vi "Test Default String Output.vi"(8 "error in (no error)":errorcluster) -> (0 "error out":errorcluster)   [LabVIEW 2016, in "UT_Formatter.lvlib"]
doc: "Template for an unit test with caraya in the \"Given, When, Then\" structure from James."
uses:
  UT_Formatter.lvlib
  Source/HSE-Logger/LogLevel.ctl
  Source/HSE-Logger/LogRecord/LogRecord.lvclass/LogRecord.ctl
  <vilib>/addons/_JKI Toolkits/Caraya/classes/Assert/Assert Equal Value_Variant.vi
  Source/HSE-Logger/Formatter/Formatter.lvclass
  <vilib>/addons/_JKI Toolkits/Caraya/classes/Test/Test.lvclass
  <vilib>/addons/_JKI Toolkits/Caraya/classes/Assert/Assert.lvclass
  Source/HSE-Logger/LogRecord/LogRecord.lvclass
  Source/HSE-Logger/hse-logger.lvlib
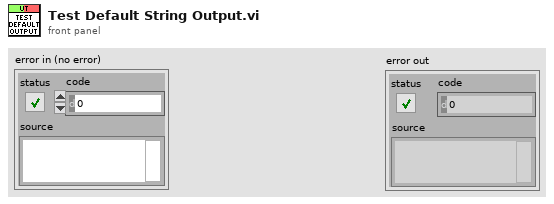
[diagram p1: front panel]
types:
  T1 = typedef "hse-logger.lvlib/LogLevel.ctl" = enum16{"DEBUG", "INFO", "WARNING", "ERROR", "CRITICAL"}
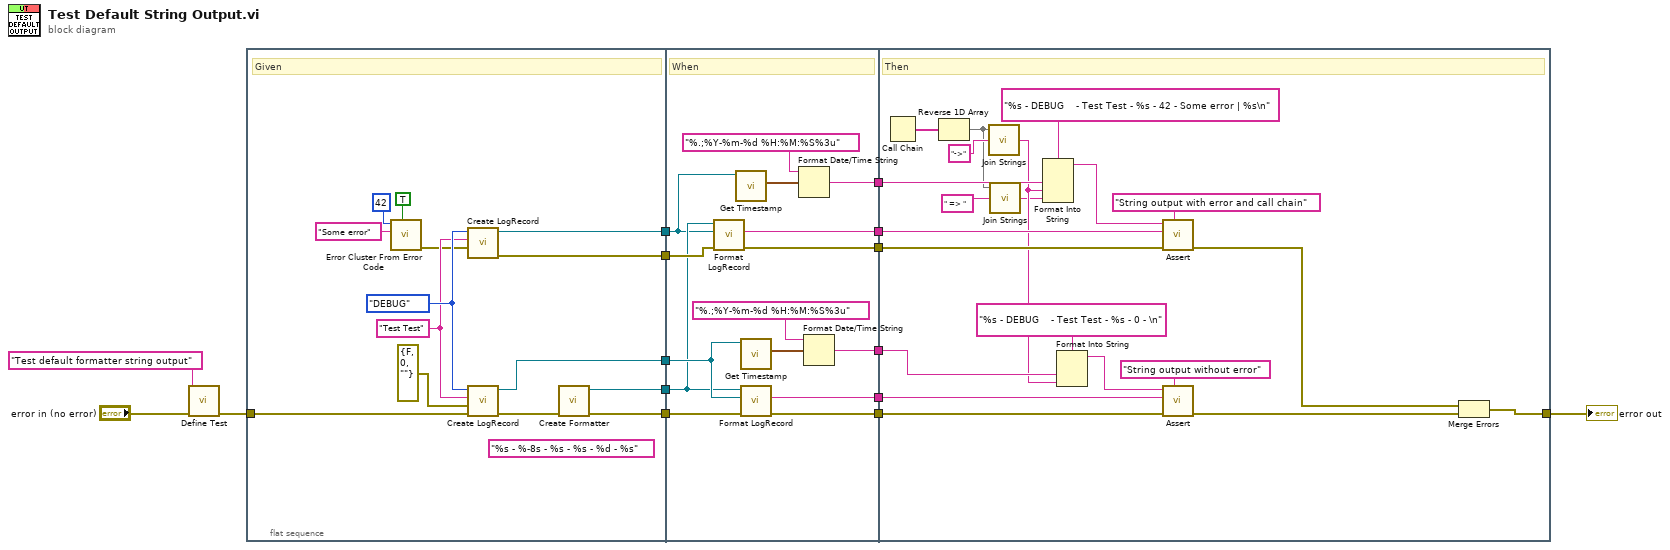
[diagram p0: block diagram]
diagram:
  n1 = call <vilib>:"Define Test.vi"("error in (no error)"="error in (no error)", "Label (VI Title)"="Test default formatter string output") -> ("error out"=w12:errorcluster)  [unwired: 8 in, 1 out]
  n2 = flat-sequence {
    tunnel: w12 -> [w29]
    tunnel: [w26] -> w15
    tunnel: [w25] -> w9
    tunnel: [w24] -> w8
    tunnel: [w18] -> w5
    tunnel: [w17] -> w4
    tunnel: w15 -> [w44]
    tunnel: [w43] -> w10
    tunnel: w9 -> [w36]
    tunnel: w8 -> [w41]
    tunnel: [w42] -> w7
    tunnel: [w38] -> w6
    tunnel: w5 -> [w37]
    tunnel: w4 -> [w32]
    tunnel: [w35] -> w3
    tunnel: [w34] -> w2
    tunnel: [w31] -> w1
    tunnel: [w65] -> w14
    tunnel: w10 -> [w63]
    tunnel: w7 -> [w61]
    tunnel: w6 -> [w58]
    tunnel: w3 -> [w56]
    tunnel: w2 -> [w57]
    tunnel: w1 -> [w54]
    frame #0 {
      (unwired) "%s - %-8s - %s - %s - %d - %s" ("Format Specifier")
      w22 = "Test Test" ("Message")
      w23 = LogLevel."DEBUG" ("Level")
      # "Given"
      n3 = call <vilib>:"Error Cluster From Error Code.vi"("show call chain? (False)"=TRUE, "error message (\"\")"="Some error" ("error message (\"\")"), "error code (0)"=42) -> ("error out"=w16:errorcluster)  [unwired: 6 in]
      n4 = call "Create LogRecord.vi"("Error to Log"=w16, "Message"=w22, "Level"=w23) -> ("error out"=w18:errorcluster, "LogRecord out"=w17:refnum<class "LogRecord.lvclass">)  [unwired: 7 in]
      n5 = call "Create LogRecord.vi"("error in"=w29, "Error to Log"=errorcluster {"status"=FALSE, "code"=0, "source"=""}, "Message"=w22, "Level"=w23) -> ("error out"=w27:errorcluster, "LogRecord out"=w24:refnum<class "LogRecord.lvclass">)  [unwired: 6 in]
      n6 = call "Create Formatter.vi"("error in"=w27) -> ("error out"=w26:errorcluster, "Formatter out"=w25:refnum<class "Formatter.lvclass">)  [unwired: 9 in]
    }
    frame #1 {
      # "When"
      n7 = call-dynamic "Format LogRecord.vi"("error in"=w37, "LogRecord"=w32, "Formatter in"=w36) -> ("error out"=w34:errorcluster, "LogLine"=w35:string)  [unwired: 7 in]
      n8 = call "Get Timestamp.vi"("LogRecord in"=w32) -> ("Created"=w33:timestamp)  [unwired: 8 in, 2 out]
      n9 = call "Get Timestamp.vi"("LogRecord in"=w41) -> ("Created"=w40:timestamp)  [unwired: 8 in, 2 out]
      n10 = call-dynamic "Format LogRecord.vi"("error in"=w44, "LogRecord"=w41, "Formatter in"=w36) -> ("error out"=w43:errorcluster, "LogLine"=w42:string)  [unwired: 7 in]
      n11 = Format Date/Time String(time format string (%c)="%.;%Y-%m-%d %H:%M:%S%3u", seconds (now)=w33) -> (date/time string=w31:string)  [unwired: 1 in]
      n12 = Format Date/Time String(time format string (%c)="%.;%Y-%m-%d %H:%M:%S%3u", seconds (now)=w40) -> (date/time string=w38:string)  [unwired: 1 in]
    }
    frame #2 {
      # "Then"
      n13 = Call Chain() -> (call chain=w46:string[])
      n14 = Reverse 1D Array(array=w46) -> (reversed array=w45:string[])
      n15 = call <vilib>:"Join Strings.vi"("Separator (,)"="->", "Strings In"=w45) -> ("String"=w49:string)  [unwired: 1 in]
      n16 = call <vilib>:"Join Strings.vi"("Separator (,)"=" => ", "Strings In"=w45) -> ("String"=w48:string)  [unwired: 1 in]
      n17 = Format Into String(format string="%s - DEBUG    - Test Test - %s - 42 - Some error | %s\n" ("Label"), w54, w49, w48) -> (resulting string=w52:string)  [unwired: 2 in, 1 out]
      n18 = Format Into String(format string="%s - DEBUG    - Test Test - %s - 0 - \n" ("Label"), w58, w49) -> (resulting string=w60:string)  [unwired: 2 in, 1 out]
      n19 = call-poly <vilib>:"Assert.vi"("Label"="String output with error and call chain", "error in (no error)"=w57, "Y"=w56, "X"=w52) -> ("error out"=w51:errorcluster)  [unwired: 6 in, 1 out]
      n20 = call-poly <vilib>:"Assert.vi"("Label"="String output without error", "error in (no error)"=w63, "Y"=w61, "X"=w60) -> ("error out"=w62:errorcluster)  [unwired: 6 in, 1 out]
      n21 = Merge Errors(w51, w62) -> (w65:errorcluster)
    }
  }
  "error out" <- w14
